vi "Coloured Column Number--Const.vi"() -> (3 "Coloured Column":i32)   [LabVIEW 2017, in "DTacq Plot Display Library.lvlib"]
uses:
  DTacq Plot Display Library.lvlib
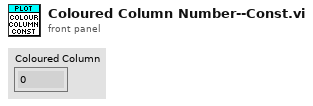
[diagram p1: front panel]
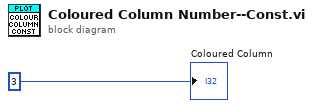
[diagram p0: block diagram]
diagram:
  "Coloured Column" <- 3 ("disabled index (col)")
